vi "Delete Selected Nodes.vi"(8 "error in (no error)":errorcluster, 11 "FSM in":refnum<class "FSM.Graph.lvclass">) -> (0 "error out":errorcluster, 3 "FSM out":refnum<class "FSM.Graph.lvclass">)   [LabVIEW 2015, in "FSM.Graph.lvclass"]
uses:
  FSM.Graph.lvclass
  FSM.Graph.lvclass/FSM.Graph.ctl
  FSM.Node/FSM.Node.lvclass/FSM.Node.ctl
  FSM.Node/Read Name.vi
  FSM.Edge/FSM.Edge.lvclass
  FSM.Node/FSM.Node.lvclass
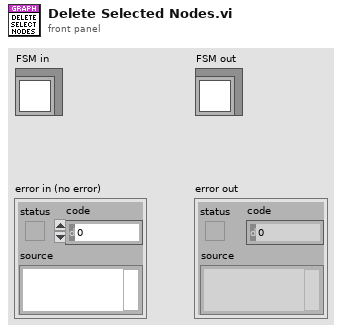
[diagram p1: front panel]
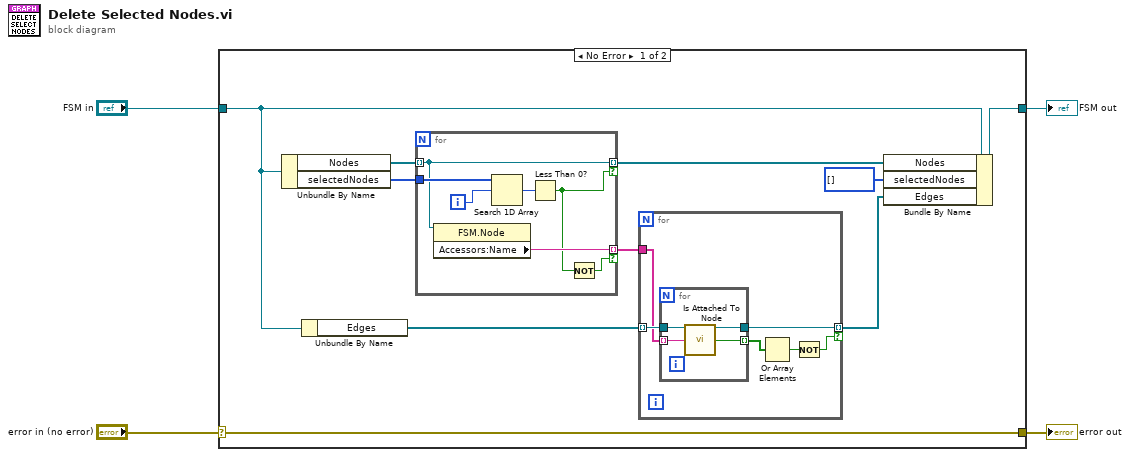
[diagram p0: block diagram]
diagram:
  n1 = case shown="No Error" "error in (no error)" {
    selector: "error in (no error)" -> [w14 w33]
    tunnel: [w14 w33] -> w3
    tunnel: [w11 w32] -> w1
    tunnel: "FSM in" -> [w8 w32]
    frame No Error {
      n2 = Unbundle By Name(w8) -> ("Nodes"=w13:refnum<class "FSM.Node.lvclass">[], "selectedNodes"=w12:i32[])
      n3 = Unbundle By Name(w8) -> ("Edges"=w7:refnum<class "FSM.Edge.lvclass">[])
      n4 = for {
        tunnel: w13 -> [w28] mode=indexing
        tunnel: w12 -> [w31]
        tunnel: [w28] -> w10 mode=indexing if=w25
        tunnel: [w27] -> w6 mode=indexing if=w26
        i -> [w30]
        n5 = property class="FSM.Node"(reference=w28) -> ("Accessors:Name"=w27:string)  [unwired: 1 in, 2 out]
        n6 = Search 1D Array(1D array=w31, element=w30) -> (index of element=w29:i32)  [unwired: 1 in]
        n7 = Less Than 0?(x=w29) -> (x < 0?=w25:bool)
        n8 = Not(x=w25) -> (.not. x?=w26:bool)
      }
      n9 = for {
        tunnel: w7 -> [w20] mode=indexing
        tunnel: w6 -> [w19]
        tunnel: [w18] -> w5 mode=indexing if=w15
        n10 = for {
          tunnel: w20 -> [w24]
          tunnel: w19 -> [w23] mode=indexing
          tunnel: [w22] -> w18
          tunnel: [w21] -> w17 mode=indexing
          n11 = call "Is Attached To Node.vi"("FSM.Edge In"=w24, "nodeName"=w23) -> ("FSM.Edge Out"=w22:refnum<class "FSM.Edge.lvclass">, "attached to"=w21:bool)  [unwired: 12 in]
        }
        n12 = Or Array Elements(Boolean array=w17) -> (logical OR=w16:bool)
        n13 = Not(x=w16) -> (.not. x?=w15:bool)
      }
      n14 = Bundle By Name(cluster=w8, "Nodes"=w10, "selectedNodes"=i32[] [], "Edges"=w5) -> (w11:refnum<class "FSM.Graph.lvclass">)
    }
    frame Error {
    }
  }
  "error out" <- w3
  "FSM out" <- w1
